vi "StartRCM_RCM.vi"(0 "Display State In":T1={"RCM File Path"=path "", "Left"=0, "Top"=0, "Font Name"="", "Font Size"=0, "Font Color"=0, "Separator Color"=9868950, "Frame Color"=9868950, "Overlay Color"=26367}, 1 "VI Refnum":refnum<vi>, 9 "Container State":T2, 11 "error in (no error)":errorcluster) -> (4 "Display State Out":T1={"RCM File Path"=path "", "Left"=0, "Top"=0, "Font Name"="", "Font Size"=0, "Font Color"=0, "Separator Color"=9868950, "Frame Color"=9868950, "Overlay Color"=26367}, 15 "error out":errorcluster)   [LabVIEW 2009, in "RCM.xctl"]
uses:
  RCM.xctl
  <vilib>/_xctls/Container State.ctl
  Ability/State_RCM.ctl
  <vilib>/_xctls/XControlSupport.lvlib
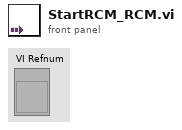
[diagram p1: front panel]
types:
  T1 = typedef "RCM.xctl/State_RCM.ctl" = cluster{"RCM File Path":path, "Left":u32, "Top":u32, "Font Name":string, "Font Size":i16, "Font Color":u32, "Separator Color":u32, "Frame Color":u32, "Overlay Color":u32}
  T2 = typedef "XControlSupport.lvlib/Container State.ctl" = cluster{"Indicator?":bool, "Run Mode?":bool, " Refnum":refnum<vi>}
  T3 = cluster{"position":cluster{"left":u32, "top":u32}, "font":cluster{"name":string, "size":i16, "color":u32}, "seperator color":u32, "frame color":u32, "overlay color":u32}
  T4 = typedef "LVRectTypeDef.ctl" = cluster{"left":i16, "top":i16, "right":i16, "bottom":i16}
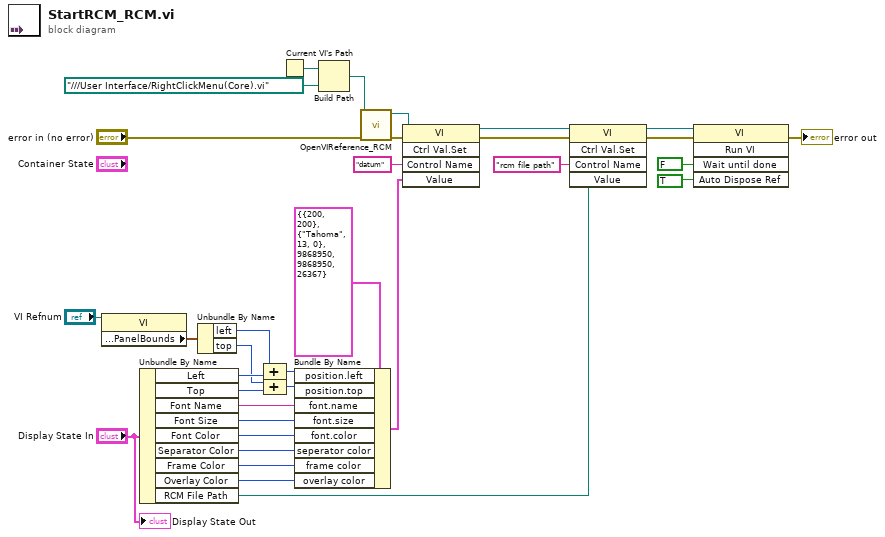
[diagram p0: block diagram]
diagram:
  n1 = property class="VI"(reference="VI Refnum") -> ("Front Panel.PanelBounds"=w5:T4)  [unwired: 1 in, 2 out]
  n2 = Unbundle By Name("Display State In") -> ("Left"=w21:u32, "Top"=w20:u32, "Font Name"=w19:string, "Font Size"=w18:i16, "Font Color"=w17:u32, "Separator Color"=w16:u32, "Frame Color"=w15:u32, "Overlay Color"=w14:u32, "RCM File Path"=w13:path)
  n3 = Unbundle By Name(w5) -> ("left"=w1:i16, "top"=w2:i16)
  n4 = Compound Arithmetic op=ADD(w1, w21) -> (w4:u32)
  n5 = Compound Arithmetic op=ADD(w2, w20) -> (w3:u32)
  n6 = Current VI's Path() -> (path=w23:path)
  n7 = Bundle By Name(cluster=T3 {"position"={"left"=200, "top"=200}, "font"={"name"="Tahoma", "size"=13, "color"=0}, "seperator color"=9868950, "frame color"=9868950, "overlay color"=26367} ("datum"), "position.left"=w4, "position.top"=w3, "font.name"=w19, "font.size"=w18, "font.color"=w17, "seperator color"=w16, "frame color"=w15, "overlay color"=w14) -> (w25:T3)
  n8 = Build Path(base path=w23, name or relative path=path "../../../User Interface/RightClickMenu(Core).vi" ("vi path")) -> (appended path=w7:path)
  n9 = call "OpenVIReference_RCM.vi"("error in (no error)"="error in (no error)", "path"=w7) -> ("error out"=w28:errorcluster, "vi reference"=w11:refnum<vi>)  [unwired: 8 in]
  n10 = invoke class="VI" method="Ctrl Val.Set"(reference=w11, error in=w28, "Control Name"="datum", "Value"=w25) -> (reference out=w10:refnum<vi>, error out=w26:errorcluster)  [unwired: 1 in, 3 out]
  n11 = invoke class="VI" method="Ctrl Val.Set"(reference=w10, error in=w26, "Control Name"="rcm file path", "Value"=w13) -> (reference out=w9:refnum<vi>, error out=w27:errorcluster)  [unwired: 1 in, 3 out]
  n12 = invoke class="VI" method="Run VI"(reference=w9, error in=w27, "Wait until done"=FALSE ("Wait Until Done"), "Auto Dispose Ref"=TRUE ("Auto Dispose Reference")) -> (error out=→"error out":errorcluster)  [unwired: 1 in, 4 out]
  "Display State Out" <- "Display State In"
